vi "capture single.vi"() -> (0 "PIXEL MAP (12bit, grayscale)":u16[][](array[numeric]) format="%x", 3 "Success":bool)   [LabVIEW 2018]
uses:
  Dll1_x64_191014_0/Dll1_x64_191014_0.lvlib
panel:
  out "query":i32
  out "block":i32
  out "read error #":i32
  out "status":string
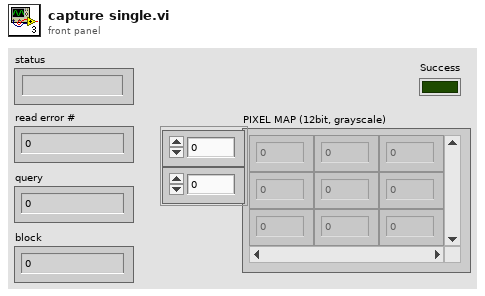
[diagram p1: front panel]
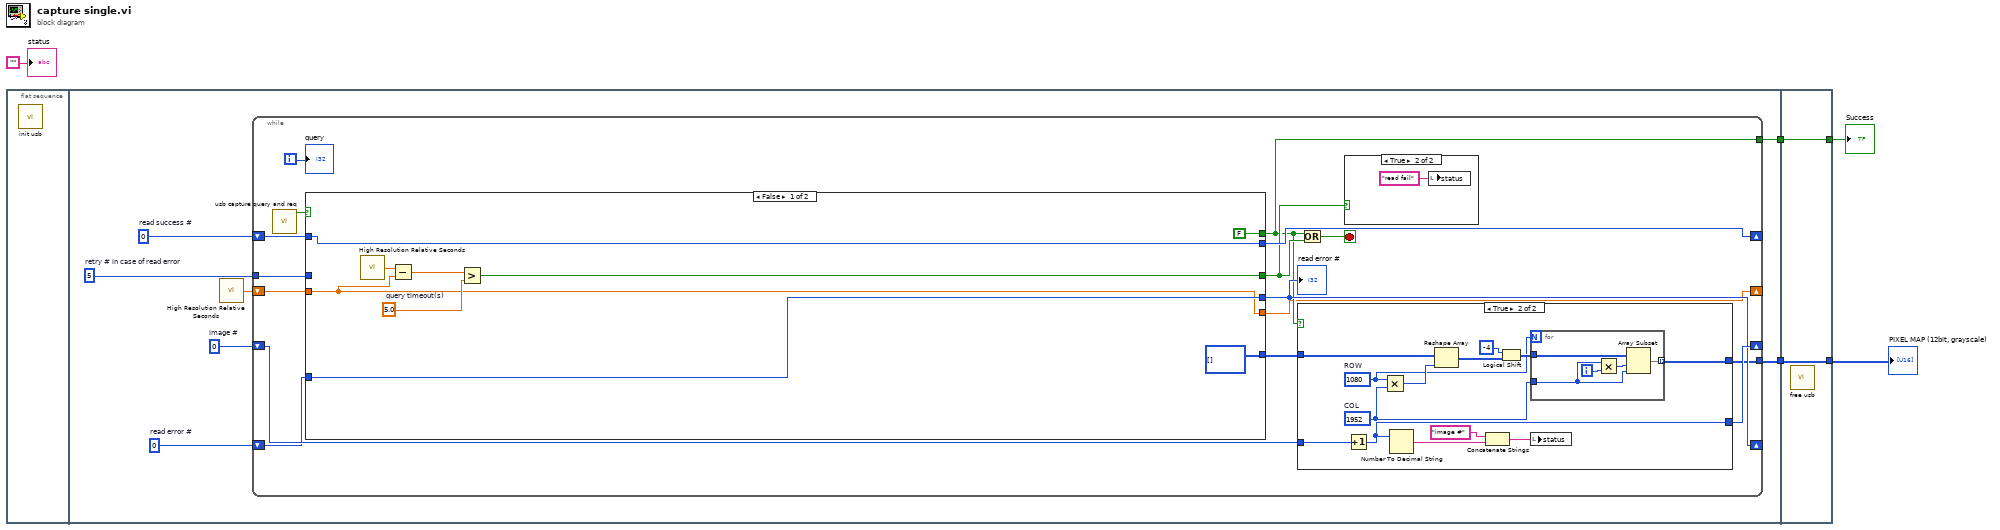
[diagram p0: block diagram]
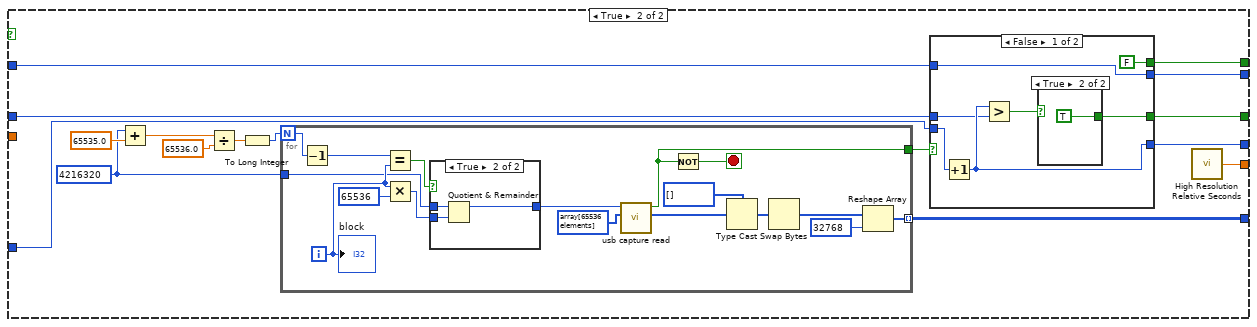
[diagram p3: hidden frame]
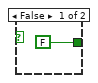
[diagram p4: hidden frame]
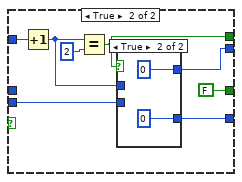
[diagram p5: hidden frame]
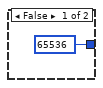
[diagram p7: hidden frame]
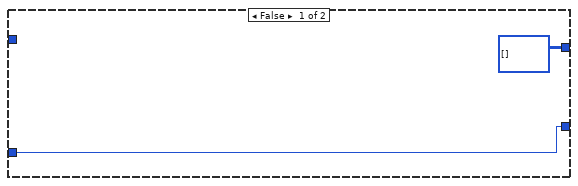
[diagram p8: hidden frame]
diagram:
  n1 = flat-sequence {
    tunnel: [w8] -> w4
    tunnel: [w7] -> w3
    tunnel: [w117] -> w1
    tunnel: w4 -> [w117]
    tunnel: [w118] -> w2
    tunnel: w3 -> [w118]
    frame #0 {
      n2 = call "init usb.vi"() -> ()  [unwired: 12 in]
    }
    frame #1 {
      w6 = 5  # retry # in case of read error
      w10 = 0  # read error #
      w11 = 0  # read success #
      w12 = 0  # image #
      n3 = call <vilib>:"High Resolution Relative Seconds.vi"() -> ("relative seconds"=w9:dbl)
      n4 = while {
        shift-right: [w25] -> _
        shift-left: w12 -> [w26]
        shift-right: [w22] -> _
        shift-left: w11 -> [w23]
        shift-right: [w19] -> _
        shift-left: w10 -> [w21]
        shift-right: [w13] -> _
        shift-left: w9 -> [w20]
        tunnel: [w18] -> w8
        tunnel: [w16] -> w7
        tunnel: w6 -> [w14]
        i -> [w28]
        stop <- w15 stop-if-true
        n5 = call "usb capture query and req.vi"() -> ("function return"=w24:bool)  [unwired: 11 in]
        n6 = case shown="False" w24 {
          tunnel: [FALSE w44] -> w16
          tunnel: [u16[][] [] w48] -> w27
          tunnel: w23 -> [w37 w46]
          tunnel: [w37 w45] -> w22
          tunnel: w21 -> [w36 w42]
          tunnel: [w36 w41] -> w19
          tunnel: w20 -> [w30 _]
          tunnel: [w31 w43] -> w17
          tunnel: w14 -> [_ w40]
          tunnel: [w30 w39] -> w13
          frame False {
            w33 = 5.0  # query timeout(s)
            n7 = call <vilib>:"High Resolution Relative Seconds.vi"() -> ("relative seconds"=w35:dbl)
            n8 = Subtract(x=w35, y=w30) -> (x-y=w34:dbl)
            n9 = Greater?(x=w34, y=w33) -> (0:w31:bool)
          }
          frame True {
            w49 = 4216320
            n10 = Add(x=w49, y=65535.0) -> (x+y=w54:dbl)
            n11 = Divide(x=w54, y=65536.0) -> (x/y=w53:dbl)
            n12 = To Long Integer(number=w53) -> (32bit integer=w50:i32)
            n13 = for {
              N: w50 -> [w88]
              tunnel: w49 -> [w86]
              tunnel: [w78] -> w48 mode=indexing
              tunnel: [w76] -> w47
              i -> [w87]
              stop <- w77 stop-if-true
              n14 = Decrement(x=w88) -> (x-1=w91:i32)
              n15 = Equal?(x=w91, y=w87) -> (x = y?=w92:bool)
              n16 = Multiply(x=w87, y=65536) -> (x*y=w89:i32)
              n17 = case shown="True" w92 {
                tunnel: [65536 ("len") w94] -> w85
                tunnel: w86 -> [_ w96]
                tunnel: w89 -> [_ w95]
                frame False {
                }
                frame True {
                  n18 = Quotient & Remainder(x=w96, y=w95) -> (x-y*floor(x/y)=w94:i32)  [unwired: 1 out]
                }
              }
              n19 = call "usb capture read.vi"("read_data"=i8[] array[65536 elements], "len"=w85) -> ("read_data out"=w82:u8[], "function return"=w76:bool)  [unwired: 8 in]
              n20 = Not(x=w76) -> (.not. x?=w77:bool)
              n21 = Type Cast(type=u16[] [], x=w82) -> (*(type *) &x=w81:u16[])
              n22 = Swap Bytes(anything=w81) -> (byte swapped=w79:u16[])
              n23 = Reshape Array(w79, 32768 ("dimension size")) -> (w78:u16[])
              "block" <- w87
            }
            n24 = case shown="False" w47 {
              tunnel: w46 -> [w61 w71]
              tunnel: [w61 w68] -> w45
              tunnel: [FALSE w67] -> w44
              tunnel: w42 -> [w57 w65]
              tunnel: [w58 FALSE] -> w43
              tunnel: [w56 w64] -> w41
              tunnel: w40 -> [w55 _]
              frame False {
                n25 = Increment(x=w57) -> (x+1=w56:i32)
                n26 = Greater?(x=w56, y=w55) -> (0:w59:bool)
                n27 = case shown="True" w59 {
                  tunnel: [FALSE TRUE] -> w58
                  frame False {
                  }
                  frame True {
                  }
                }
              }
              frame True {
                n28 = Increment(x=w71) -> (x+1=w69:i32)
                n29 = Equal?(x=w69, y=2) -> (x = y?=w67:bool)
                n30 = case shown="True" w67 {
                  tunnel: w69 -> [w73 _]
                  tunnel: [w73 0] -> w68
                  tunnel: w65 -> [w72 _]
                  tunnel: [w72 0] -> w64
                  frame False {
                  }
                  frame True {
                  }
                }
              }
            }
            n31 = call <vilib>:"High Resolution Relative Seconds.vi"() -> ("relative seconds"=w39:dbl)
          }
        }
        "read error #" <- w19
        n32 = case shown="True" w16 {
          tunnel: w27 -> [_ w100]
          tunnel: w26 -> [w98 w111]
          tunnel: [w98 w107] -> w25
          tunnel: [u16[][] [] w99] -> w18
          frame False {
          }
          frame True {
            w102 = 1952  # COL
            w103 = 1080  # ROW
            n33 = Increment(x=w111) -> (x+1=w107:i32)
            n34 = Multiply(x=w103, y=w102) -> (x*y=w106:i32)
            n35 = Number To Decimal String(number=w107) -> (decimal integer string=w109:string)  [unwired: 1 in]
            n36 = Reshape Array(w100, w106) -> (w105:u16[])
            n37 = Concatenate Strings("image #" ("string"), w109) -> (w110:string)
            n38 = Logical Shift(y=i16 -4, x=w105) -> (x << y=w104:u16[])
            n39 = for {
              N: w103 -> [_]
              tunnel: w104 -> [w115]
              tunnel: [w113] -> w99 mode=indexing
              tunnel: w102 -> [w112]
              i -> [w116]
              n40 = Multiply(x=w112, y=w116) -> (x*y=w114:i32)
              n41 = Array Subset(array=w115, index=w114, length=w112) -> (w113:u16[])
            }
            n42 = local write "status"(w110) -> ()
          }
        }
        n43 = Or(x=w16, y=w17) -> (x .or. y?=w15:bool)
        n44 = case shown="True" w17 {
          frame False {
          }
          frame True {
            n45 = local write "status"("read fail" ("string")) -> ()
          }
        }
        "query" <- w28
      }
    }
    frame #2 {
      n46 = call "free usb.vi"() -> ()  [unwired: 12 in]
    }
  }
  "PIXEL MAP (12bit, grayscale)" <- w1
  "Success" <- w2
  "status" <- ""
